vi "getRunItem.vi"(8 "error in (no error)":errorcluster, 11 "Run in":refnum<k24>) -> (0 "error out":errorcluster, 1 "Style out":refnum<class "Style.lvclass">, 2 "Paragraph":refnum<k24>, 3 "Run out":refnum<k24>)   [LabVIEW 2017, in "xwpfReader.lvclass"]
uses:
  xwpfReader.lvclass
  Styles/Style/Style.lvclass
  C:/Users/Neo/Desktop/Dev_Tools_BR/LabVIEW_NPOI/src/lib/NPOI 2.1.1/NPOI.OOXML.dll
  lib/NPOI 2.1.1/NPOI.OOXML.dll
  Styles/Font--cluster.ctl
  Styles/Underline--ring.ctl
  Styles/Alignment--ring.ctl
  Styles/Styles.lvlib
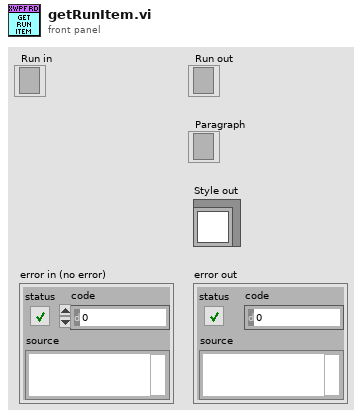
[diagram p1: front panel]
types:
  T1 = typedef "Styles.lvlib/Font--cluster.ctl" = cluster{"Name":string, "Size":i32, "Bold":bool, "Italic":bool, "Underline":T2, "Strike":bool, "Color":u32, "Alignment":T3}
  T2 = typedef "Styles.lvlib/Underline--ring.ctl" = i32
  T3 = typedef "Styles.lvlib/Alignment--ring.ctl" = i32
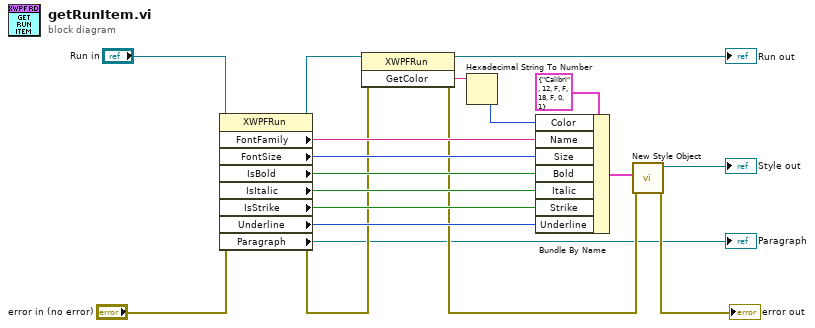
[diagram p0: block diagram]
diagram:
  n1 = property class="XWPFRun"(reference="Run in", error in="error in (no error)") -> (reference out=w9:refnum<k24>, error out=w3:errorcluster, "FontFamily"=w10:string, "FontSize"=w11:i32, "IsBold"=w12:bool, "IsItalic"=w13:bool, "IsStrike"=w14:bool, "Underline"=w15:i32, "Paragraph"=→"Paragraph":refnum<k24>)
  n2 = invoke class="XWPFRun" method="GetColor"(reference=w9, error in=w3) -> (reference out=→"Run out":refnum<k24>, error out=w2:errorcluster, "GetColor"=w5:string)  [unwired: 1 in]
  n3 = Hexadecimal String To Number(string=w5) -> (number=w4:u32)  [unwired: 2 in, 1 out]
  n4 = Bundle By Name(cluster=T1 {"Name"="Calibri", "Size"=12, "Bold"=FALSE, "Italic"=FALSE, "Underline"=18, "Strike"=FALSE, "Color"=0, "Alignment"=1} ("Font"), "Color"=w4, "Name"=w10, "Size"=w11, "Bold"=w12, "Italic"=w13, "Strike"=w14, "Underline"=w15) -> (w17:T1)
  n5 = call "New Style Object.vi"("error in (no error)"=w2, "Font"=w17) -> ("error out"=→"error out":errorcluster, "Style out"=→"Style out":refnum<class "Style.lvclass">)  [unwired: 8 in]
